vi "Get Thing Shadow Details.vi"(8 "error in (no error)":errorcluster, 11 "Thing Shadow in":refnum<class "Thing Shadow.lvclass">) -> (0 "error out":errorcluster, 1 "Reported State":T1[](array[typedef]), 2 "Desired State":T1[](array[typedef]), 3 "Thing Shadow out":refnum<class "Thing Shadow.lvclass">, 4 "Version":i32, 5 "Raw JSON":string)   [LabVIEW 2015, in "NI_AWS_IoT.lvlib" / "Thing Shadow.lvclass"]
uses:
  Thing Shadow.lvclass
  JSON Parsing/Name-Value with Type.ctl
  JSON Parsing/Name Value Pair.ctl
  JSON Parsing/JSON Type.ctl
  Core/HTTP Request/Request Options.ctl
  Core/HTTP Request/Name Value Pair.ctl
  Core/HTTP Request/Region handling.ctl
  Core/HTTP Request/URL formatting.ctl
  Thing Shadow.lvclass/Thing Shadow.ctl
  Read Thing Name.vi
  Core/HTTP Request/HTTP Request.lvclass
  NI_AWS_IoT.lvlib
  JSON Parsing/NI_JSON Parsing.lvlib
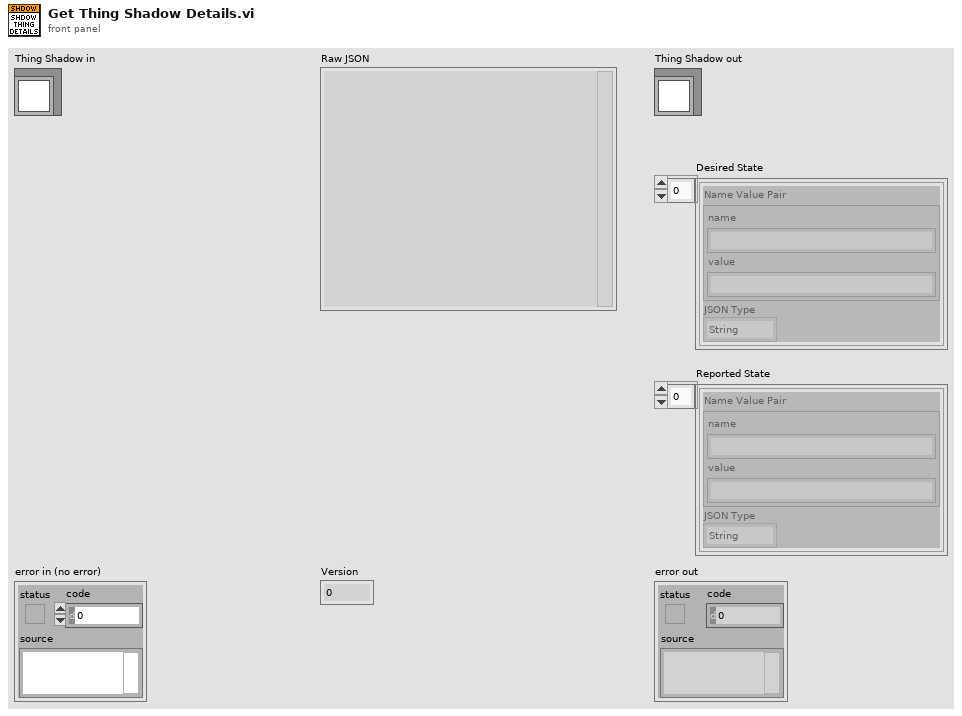
[diagram p1: front panel]
types:
  T1 = typedef "NI_JSON Parsing.lvlib/Name-Value with Type.ctl" = cluster{"Name Value Pair":T2, "JSON Type":T3}
  T2 = typedef "NI_JSON Parsing.lvlib/Name Value Pair.ctl" = cluster{"name":string, "value":string}
  T3 = typedef "NI_JSON Parsing.lvlib/JSON Type.ctl" = enum16{"String", "Numeric", "Boolean"}
  T4 = typedef "NI_AWS_Core.lvlib/HTTP Request.lvclass/Name Value Pair.ctl" = cluster{"name":string, "value":string}
  T5 = typedef "NI_AWS_Core.lvlib/HTTP Request.lvclass/Request Options.ctl" = cluster{"request headers":T4[], "request parameters":T4[], "request body":string, "region handling":T6, "URL formatting":T7}
  T6 = typedef "NI_AWS_Core.lvlib/HTTP Request.lvclass/Region handling.ctl" = enum16{"use region everywhere", "use region (authentication only)", "use region (URL only)", "ignore region everwhere"}
  T7 = typedef "NI_AWS_Core.lvlib/HTTP Request.lvclass/URL formatting.ctl" = enum16{"region-", "region."}
  T8 = typedef "NI_AWS_Core.lvlib/HTTP Request.lvclass/Response.ctl" = cluster{"Headers":string, "Body":string}
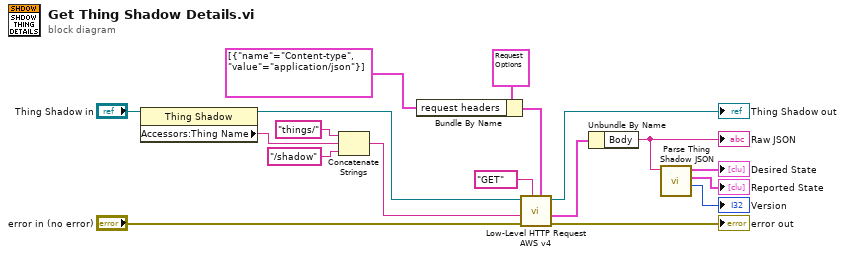
[diagram p0: block diagram]
diagram:
  n1 = property class="Thing Shadow"(reference="Thing Shadow in") -> (reference out=w7:refnum<class "Thing Shadow.lvclass">, "Accessors:Thing Name"=w6:string)  [unwired: 1 in, 1 out]
  n2 = Concatenate Strings("things/" ("string"), w6, "/shadow" ("string")) -> (w12:string)
  n3 = Bundle By Name(cluster=T5 {"request headers"=[], "request parameters"=[], "request body"="", "region handling"=enum."use region everywhere", "URL formatting"=enum."region."} ("Request Options"), "request headers"=T4[] [{"name"="Content-type", "value"="application/json"}]) -> (w13:T5)
  n4 = call "Low-Level HTTP Request AWS v4.vi"("Request Options"=w13, "HTTP-Verb"="GET", "error in (no error)"="error in (no error)", "URL Suffix"=w12, "AWS Core in"=w7) -> ("error out"=→"error out":errorcluster, "Response"=w9:T8, "AWS Core out"=→"Thing Shadow out":refnum<class "Thing Shadow.lvclass">)  [unwired: 3 in, 1 out]
  n5 = Unbundle By Name(w9) -> ("Body"=w4:string)
  "Raw JSON" <- w4
  n6 = call "Parse Thing Shadow JSON.vi"("JSON"=w4) -> ("Version"=→"Version":i32, "Reported State"=→"Reported State":T1[], "Desired State"=→"Desired State":T1[])  [unwired: 8 in]
